vi "Configure Chevelle JESD TX.vi"(0 "fpga ref in":T1, 11 "error in (no error)":errorcluster) -> (4 "fpga ref out":T1, 15 "error out":errorcluster)   [LabVIEW 2019]
uses:
  TypeDefs/Blank FPGA Reference.ctl
  TypeDefs/TX FPGA Reference.ctl
  <vilib>/rvi/errors/niLvFpgaAdjustHostInterfaceError.vi
  <vilib>/rvi/interface/nirviReadWriteControl/nirviReadWriteControl.xnode
  <vilib>/rvi/interface/Simulation/niFpgaSimulationCallBeginRW.vi
  NiFpgaLv.dll
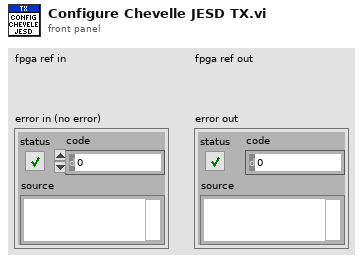
[diagram p1: front panel]
types:
  T1 = typedef "Blank FPGA Reference.ctl" = refnum<k20>
  T2 = typedef "TX FPGA Reference.ctl" = refnum<k20>
  T3 = cluster{"reset":bool, "gtx enable":bool, "jesd enable":bool, "sw sync":bool, "gtx post cursor":fxp<+,5,5>, "gtx pre cursor":fxp<+,5,5>, "gtx diff control":fxp<+,4,4>, "clock enable":bool, "lmfc delay":fxp<+,5,5>, "sysref enable":bool, "sync enable":bool, "trig7 listen":bool, "trig7 invert":bool, "clear data in error":bool}
  T4 = cluster{"gtx active":bool, "jesd active":bool, "lane sync req":bool, "lanes synced":bool, "lanes aligned":bool, "qpll locked":bool, "qpll ref lost":bool, "mgt ref clocks locked":bool, "mgt ref clock valid":bool, "data error":bool}
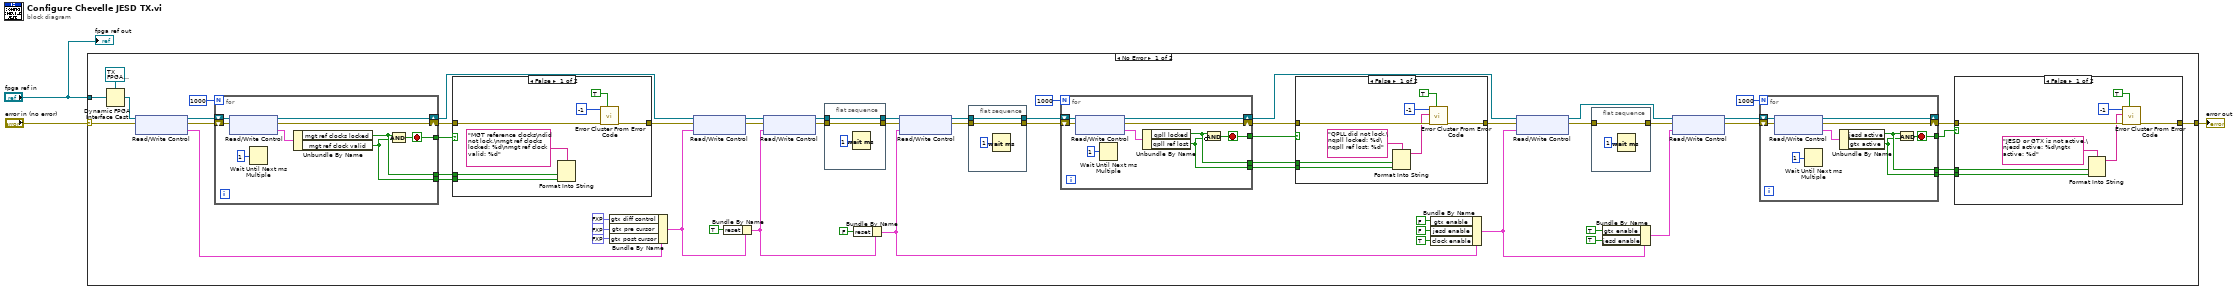
[diagram p0: block diagram]
diagram:
  n1 = case shown="No Error" "error in (no error)" {
    selector: "error in (no error)" -> [w27 w122]
    tunnel: "fpga ref in" -> [w43 _]
    tunnel: [w30 w122] -> w3
    frame No Error {
      n2 = Dynamic FPGA Interface Cast(Session In=T2 refnum ("Refnum in"), Type=w43) -> (Session Out=w29:T2)
      n3 = xnode "Read/Write Control"("FPGA VI Reference In"=w29, "error in"=w27) -> ("FPGA VI Reference Out"=w28:T2, "error out"=w26:errorcluster, "txjesd.control"=w25:T3)
      n4 = for {
        N: 1000 -> [_]
        shift-right: [w86] -> w53
        shift-left: w28 -> [w84]
        shift-right: [w85] -> w34
        shift-left: w26 -> [w83]
        tunnel: [w81] -> w35
        tunnel: [w79] -> w9
        tunnel: [w78] -> w8
        stop <- w81 stop-if-true
        n5 = xnode "Read/Write Control"("FPGA VI Reference In"=w84, "error in"=w83) -> ("FPGA VI Reference Out"=w86:T2, "error out"=w85:errorcluster, "txjesd.status"=w80:T4)
        n6 = Wait Until Next ms Multiple(millisecond multiple=u32 1) -> ()  [unwired: 1 out]
        n7 = Unbundle By Name(w80) -> ("mgt ref clocks locked"=w79:bool, "mgt ref clock valid"=w78:bool)
        n8 = Compound Arithmetic op=AND(w79, w78) -> (w81:bool)
      }
      n9 = case shown="False" w35 {
        tunnel: w34 -> [w93 w94]
        tunnel: [w92 w94] -> w33
        tunnel: w9 -> [w88 _]
        tunnel: w8 -> [w87 _]
        frame False {
          n10 = Format Into String(format string="MGT reference clocks\ndid not lock.\nmgt ref clocks locked: %d\nmgt ref clock valid: %d", w88, w87) -> ()  [unwired: 2 in, 2 out]
          n11 = call <vilib>:"Error Cluster From Error Code.vi"("show call chain? (False)"=TRUE ("is warning? (False)"), "error in (no error)"=w93, "error code (0)"=-1) -> ("error out"=w92:errorcluster)  [unwired: 6 in]
        }
        frame True {
        }
      }
      n12 = Bundle By Name(cluster=w25, "gtx diff control"=fxp<+,4,4> 15.0 ("txjesd.gtx diff control"), "gtx pre cursor"=fxp<+,5,5> 0.0 ("txjesd.gtx pre cursor"), "gtx post cursor"=fxp<+,5,5> 0.0 ("txjesd.gtx post cursor")) -> (w21:T3)
      n13 = xnode "Read/Write Control"("FPGA VI Reference In"=w53, "error in"=w33, "txjesd.control"=w21) -> ("FPGA VI Reference Out"=w54:T2, "error out"=w55:errorcluster)
      n14 = Bundle By Name(cluster=w21, "reset"=TRUE ("txjesd.reset")) -> (w16:T3)
      n15 = xnode "Read/Write Control"("FPGA VI Reference In"=w54, "error in"=w55, "txjesd.control"=w16) -> ("FPGA VI Reference Out"=w49:T2, "error out"=w50:errorcluster)
      n16 = flat-sequence {
        tunnel: w49 -> [w67]
        tunnel: w50 -> [w66]
        tunnel: [w67] -> w46
        tunnel: [w66] -> w45
        frame #0 {
          n17 = Wait (ms)(milliseconds to wait=u32 1) -> ()  [unwired: 1 out]
        }
      }
      n18 = Bundle By Name(cluster=w16, "reset"=FALSE ("txjesd.reset")) -> (w15:T3)
      n19 = xnode "Read/Write Control"("FPGA VI Reference In"=w46, "error in"=w45, "txjesd.control"=w15) -> ("FPGA VI Reference Out"=w47:T2, "error out"=w48:errorcluster)
      n20 = flat-sequence {
        tunnel: w47 -> [w64]
        tunnel: w48 -> [w63]
        tunnel: [w64] -> w56
        tunnel: [w63] -> w57
        frame #0 {
          n21 = Wait (ms)(milliseconds to wait=u32 1) -> ()  [unwired: 1 out]
        }
      }
      n22 = for {
        N: 1000 -> [_]
        shift-right: [w77] -> w42
        shift-left: w56 -> [w75]
        shift-right: [w76] -> w37
        shift-left: w57 -> [w74]
        tunnel: [w72] -> w38
        tunnel: [w70] -> w7
        tunnel: [w69] -> w6
        stop <- w72 stop-if-true
        n23 = xnode "Read/Write Control"("FPGA VI Reference In"=w75, "error in"=w74) -> ("FPGA VI Reference Out"=w77:T2, "error out"=w76:errorcluster, "txjesd.status"=w71:T4)
        n24 = Wait Until Next ms Multiple(millisecond multiple=u32 1) -> ()  [unwired: 1 out]
        n25 = Unbundle By Name(w71) -> ("qpll locked"=w70:bool, "qpll ref lost"=w69:bool)
        n26 = Compound Arithmetic op=AND(w70, invert w69) -> (w72:bool)
      }
      n27 = case shown="False" w38 {
        tunnel: w37 -> [w102 w103]
        tunnel: [w101 w103] -> w36
        tunnel: w7 -> [w96 _]
        tunnel: w6 -> [w95 _]
        frame False {
          n28 = Format Into String(format string="QPLL did not lock.\nqpll locked: %d\nqpll ref lost: %d", w96, w95) -> (resulting string=w97:string)  [unwired: 2 in, 1 out]
          n29 = call <vilib>:"Error Cluster From Error Code.vi"("show call chain? (False)"=TRUE ("is warning? (False)"), "error in (no error)"=w102, "error message (\"\")"=w97, "error code (0)"=-1) -> ("error out"=w101:errorcluster)  [unwired: 5 in]
        }
        frame True {
        }
      }
      n30 = Bundle By Name(cluster=w15, "gtx enable"=FALSE ("txjesd.reset"), "jesd enable"=FALSE, "clock enable"=TRUE) -> (w11:T3)
      n31 = xnode "Read/Write Control"("FPGA VI Reference In"=w42, "error in"=w36, "txjesd.control"=w11) -> ("FPGA VI Reference Out"=w41:T2, "error out"=w40:errorcluster)
      n32 = flat-sequence {
        tunnel: w40 -> [w61]
        tunnel: [w61] -> w39
        frame #0 {
          n33 = Wait (ms)(milliseconds to wait=u32 1) -> ()  [unwired: 1 out]
        }
      }
      n34 = Bundle By Name(cluster=w11, "gtx enable"=TRUE ("txjesd.reset"), "jesd enable"=TRUE) -> (w10:T3)
      n35 = xnode "Read/Write Control"("FPGA VI Reference In"=w41, "error in"=w39, "txjesd.control"=w10) -> ("FPGA VI Reference Out"=w58:T2, "error out"=w59:errorcluster)
      n36 = for {
        N: 1000 -> [_]
        shift-right: [w112] -> _
        shift-left: w58 -> [w110]
        shift-right: [w111] -> w31
        shift-left: w59 -> [w109]
        tunnel: [w107] -> w32
        tunnel: [w105] -> w5
        tunnel: [w104] -> w4
        stop <- w107 stop-if-true
        n37 = xnode "Read/Write Control"("FPGA VI Reference In"=w110, "error in"=w109) -> ("FPGA VI Reference Out"=w112:T2, "error out"=w111:errorcluster, "txjesd.status"=w106:T4)
        n38 = Wait Until Next ms Multiple(millisecond multiple=u32 1) -> ()  [unwired: 1 out]
        n39 = Unbundle By Name(w106) -> ("jesd active"=w105:bool, "gtx active"=w104:bool)
        n40 = And(x=w105, y=w104) -> (x .and. y?=w107:bool)
      }
      n41 = case shown="False" w32 {
        tunnel: w31 -> [w120 w121]
        tunnel: [w119 w121] -> w30
        tunnel: w5 -> [w114 _]
        tunnel: w4 -> [w113 _]
        frame False {
          n42 = Format Into String(format string="JESD or GTX is not active.\njesd active: %d\ngtx active: %d", w114, w113) -> (resulting string=w115:string)  [unwired: 2 in, 1 out]
          n43 = call <vilib>:"Error Cluster From Error Code.vi"("show call chain? (False)"=TRUE ("is warning? (False)"), "error in (no error)"=w120, "error message (\"\")"=w115, "error code (0)"=-1) -> ("error out"=w119:errorcluster)  [unwired: 5 in]
        }
        frame True {
        }
      }
    }
    frame Error {
    }
  }
  "error out" <- w3
  "fpga ref out" <- "fpga ref in"
